vi "pathplan_vertices_send.vi"(1 "vertices":dbl[][](array[numeric]), 2 "distance_all":dbl, 4 "speed_max":dbl, 5 "写入串口":refnum<visa-resource-name>) -> (20 "路径规划数据写入缓冲区":string)   [LabVIEW 2016]
uses:
  <vilib>/imath/engines/lvmath2/RunTimeEngine/NodeEndStatement/NIMS_NodeEndStatement_Output.vi
  <instcachedir>/0/NIMS_NodeEndStatement_Output_53EC0D466D134D7ABD903AC30B43404B.lvgen/NIMS_NodeEndStatement_Output_53EC0D466D134D7ABD903AC30B43404B_011.vi
  <instcachedir>/0/NIMS_NodeEndStatement_Output_53EC0D466D134D7ABD903AC30B43404B.lvgen/NIMS_NodeEndStatement_Output_53EC0D466D134D7ABD903AC30B43404B_015.vi
  <vilib>/imath/engines/lvmath2/RunTimeEngine/ErrorHandling/NIMS_Finalize Error.vi
  <vilib>/imath/engines/lvmath2/RunTimeEngine/IndexRead/NIMS M($,S).vi
  <instcachedir>/0/NIMS M($,S)_3E5749BBB62E49528D4765A77F1F6D98.lvgen/NIMS M($,S)_3E5749BBB62E49528D4765A77F1F6D98_000.vi
  <vilib>/imath/engines/lvmath2/RunTimeEngine/ArithmeticOperatorToken/NIMS_ArithmeticOperator_minus.vi
  <instcachedir>/0/NIMS_ArithmeticOperator_minus_E3B65B1D26A44BB184AFDC5B3F458E3D.lvgen/NIMS_ArithmeticOperator_minus_E3B65B1D26A44BB184AFDC5B3F458E3D_017.vi
  <vilib>/imath/engines/lvmath2/RunTimeEngine/BuiltInFunctions/norm/NIMS_norm(GV,DBL).vi
  <instcachedir>/0/NIMS_norm(GV,DBL)_1268AFF3C646412B8C6EA3CE75D09042.lvgen/NIMS_norm(GV,DBL)_1268AFF3C646412B8C6EA3CE75D09042_000.vi
  <vilib>/imath/engines/lvmath2/RunTimeEngine/ErrorHandling/NIMS_Create Error From Enums.vi
  <vilib>/imath/engines/lvmath2/RunTimeEngine/RowToken/NIMS_RowToken_M_CV.vi
  <instcachedir>/0/NIMS_RowToken_M_CV_FA79F1D1D17D44459F3ED8E09EE8B625.lvgen/NIMS_RowToken_M_CV_FA79F1D1D17D44459F3ED8E09EE8B625_003.vi
  <vilib>/imathl/engines/lvmath/Functions/Error Handling/Create Error.vi
  <vilib>/imath/engines/lvmath2/RunTimeEngine/IndexRead/NIMS M($,R2).vi
  <instcachedir>/0/NIMS M($,R2)_D9380E19261A4ADFB2D364AF6959C6EF.lvgen/NIMS M($,R2)_D9380E19261A4ADFB2D364AF6959C6EF_001.vi
  <instcachedir>/0/NIMS_RowToken_M_CV_FA79F1D1D17D44459F3ED8E09EE8B625.lvgen/NIMS_RowToken_M_CV_FA79F1D1D17D44459F3ED8E09EE8B625_000.vi
  <vilib>/imath/engines/lvmath2/RunTimeEngine/BuiltInFunctions/size/NIMS_I32=size(GM,I32).vi
  <instcachedir>/0/NIMS_I32=size(GM,I32)_122058B1B3294FAEA5DC209B92B394E4.lvgen/NIMS_I32=size(GM,I32)_122058B1B3294FAEA5DC209B92B394E4_004.vi
  <vilib>/imath/engines/lvmath2/RunTimeEngine/RangeToken/NIMS_Range_R2 - Integer.vi
  <instcachedir>/0/NIMS_Range_R2 - Integer_89B873E74E6E489885E44F751DD9C6BF.lvgen/NIMS_Range_R2 - Integer_89B873E74E6E489885E44F751DD9C6BF_000.vi
  <vilib>/imath/engines/lvmath2/RunTimeEngine/CommandStatement/MC_CommandStatement_break.vi
  <instcachedir>/0/NIMS_ArithmeticOperator_minus_E3B65B1D26A44BB184AFDC5B3F458E3D.lvgen/NIMS_ArithmeticOperator_minus_E3B65B1D26A44BB184AFDC5B3F458E3D_003.vi
  <vilib>/imath/engines/lvmath2/RunTimeEngine/VariableToken/NIMS_VariableToken_CondDefined.vi
  <instcachedir>/0/NIMS_VariableToken_CondDefined_06E9DA95BD4D46A6BA55EC651A891960.lvgen/NIMS_VariableToken_CondDefined_06E9DA95BD4D46A6BA55EC651A891960_009.vi
  <vilib>/imath/engines/lvmath/Functions/Error Handling/MergeErrorsWrapper.vi
  <instcachedir>/0/NIMS_NodeEndStatement_Output_53EC0D466D134D7ABD903AC30B43404B.lvgen/NIMS_NodeEndStatement_Output_53EC0D466D134D7ABD903AC30B43404B_005.vi
  <instcachedir>/0/NIMS_NodeEndStatement_Output_53EC0D466D134D7ABD903AC30B43404B.lvgen/NIMS_NodeEndStatement_Output_53EC0D466D134D7ABD903AC30B43404B_010.vi
  <vilib>/imath/engines/lvmath2/RunTimeEngine/BuiltInFunctions/length/NIMS_length(GM).vi
  <instcachedir>/0/NIMS_length(GM)_47CEC356FCE0482D9BA47DC61C99F2C7.lvgen/NIMS_length(GM)_47CEC356FCE0482D9BA47DC61C99F2C7_000.vi
  <instcachedir>/0/NIMS_ArithmeticOperator_minus_E3B65B1D26A44BB184AFDC5B3F458E3D.lvgen/NIMS_ArithmeticOperator_minus_E3B65B1D26A44BB184AFDC5B3F458E3D_012.vi
  <vilib>/imath/engines/lvmath2/RunTimeEngine/IndexRead/NIMS V(S).vi
  <instcachedir>/0/NIMS V(S)_0488751826AF41519A22953C041130DC.lvgen/NIMS V(S)_0488751826AF41519A22953C041130DC_000.vi
  <instcachedir>/0/NIMS V(S)_0488751826AF41519A22953C041130DC.lvgen/NIMS V(S)_0488751826AF41519A22953C041130DC_002.vi
  <vilib>/imath/engines/lvmath2/RunTimeEngine/BuiltInFunctions/dot/NIMS_dot(GV,GV).vi
  <instcachedir>/0/NIMS_dot(GV,GV)_B9FAA411F4494E9B94D442721014A3FA.lvgen/NIMS_dot(GV,GV)_B9FAA411F4494E9B94D442721014A3FA_000.vi
  <instcachedir>/0/NIMS_NodeEndStatement_Output_53EC0D466D134D7ABD903AC30B43404B.lvgen/NIMS_NodeEndStatement_Output_53EC0D466D134D7ABD903AC30B43404B_009.vi
panel:
  out "队列中元素数量":i32
  out "元素":cluster{sgl, sgl, sgl, bool}
  out "vertices_set":i32[][](array[numeric])
  out "angle_send":dbl[](array[numeric])
  out "vertices_send":dbl[](array[numeric])
  out "speed_send":dbl[](array[numeric])
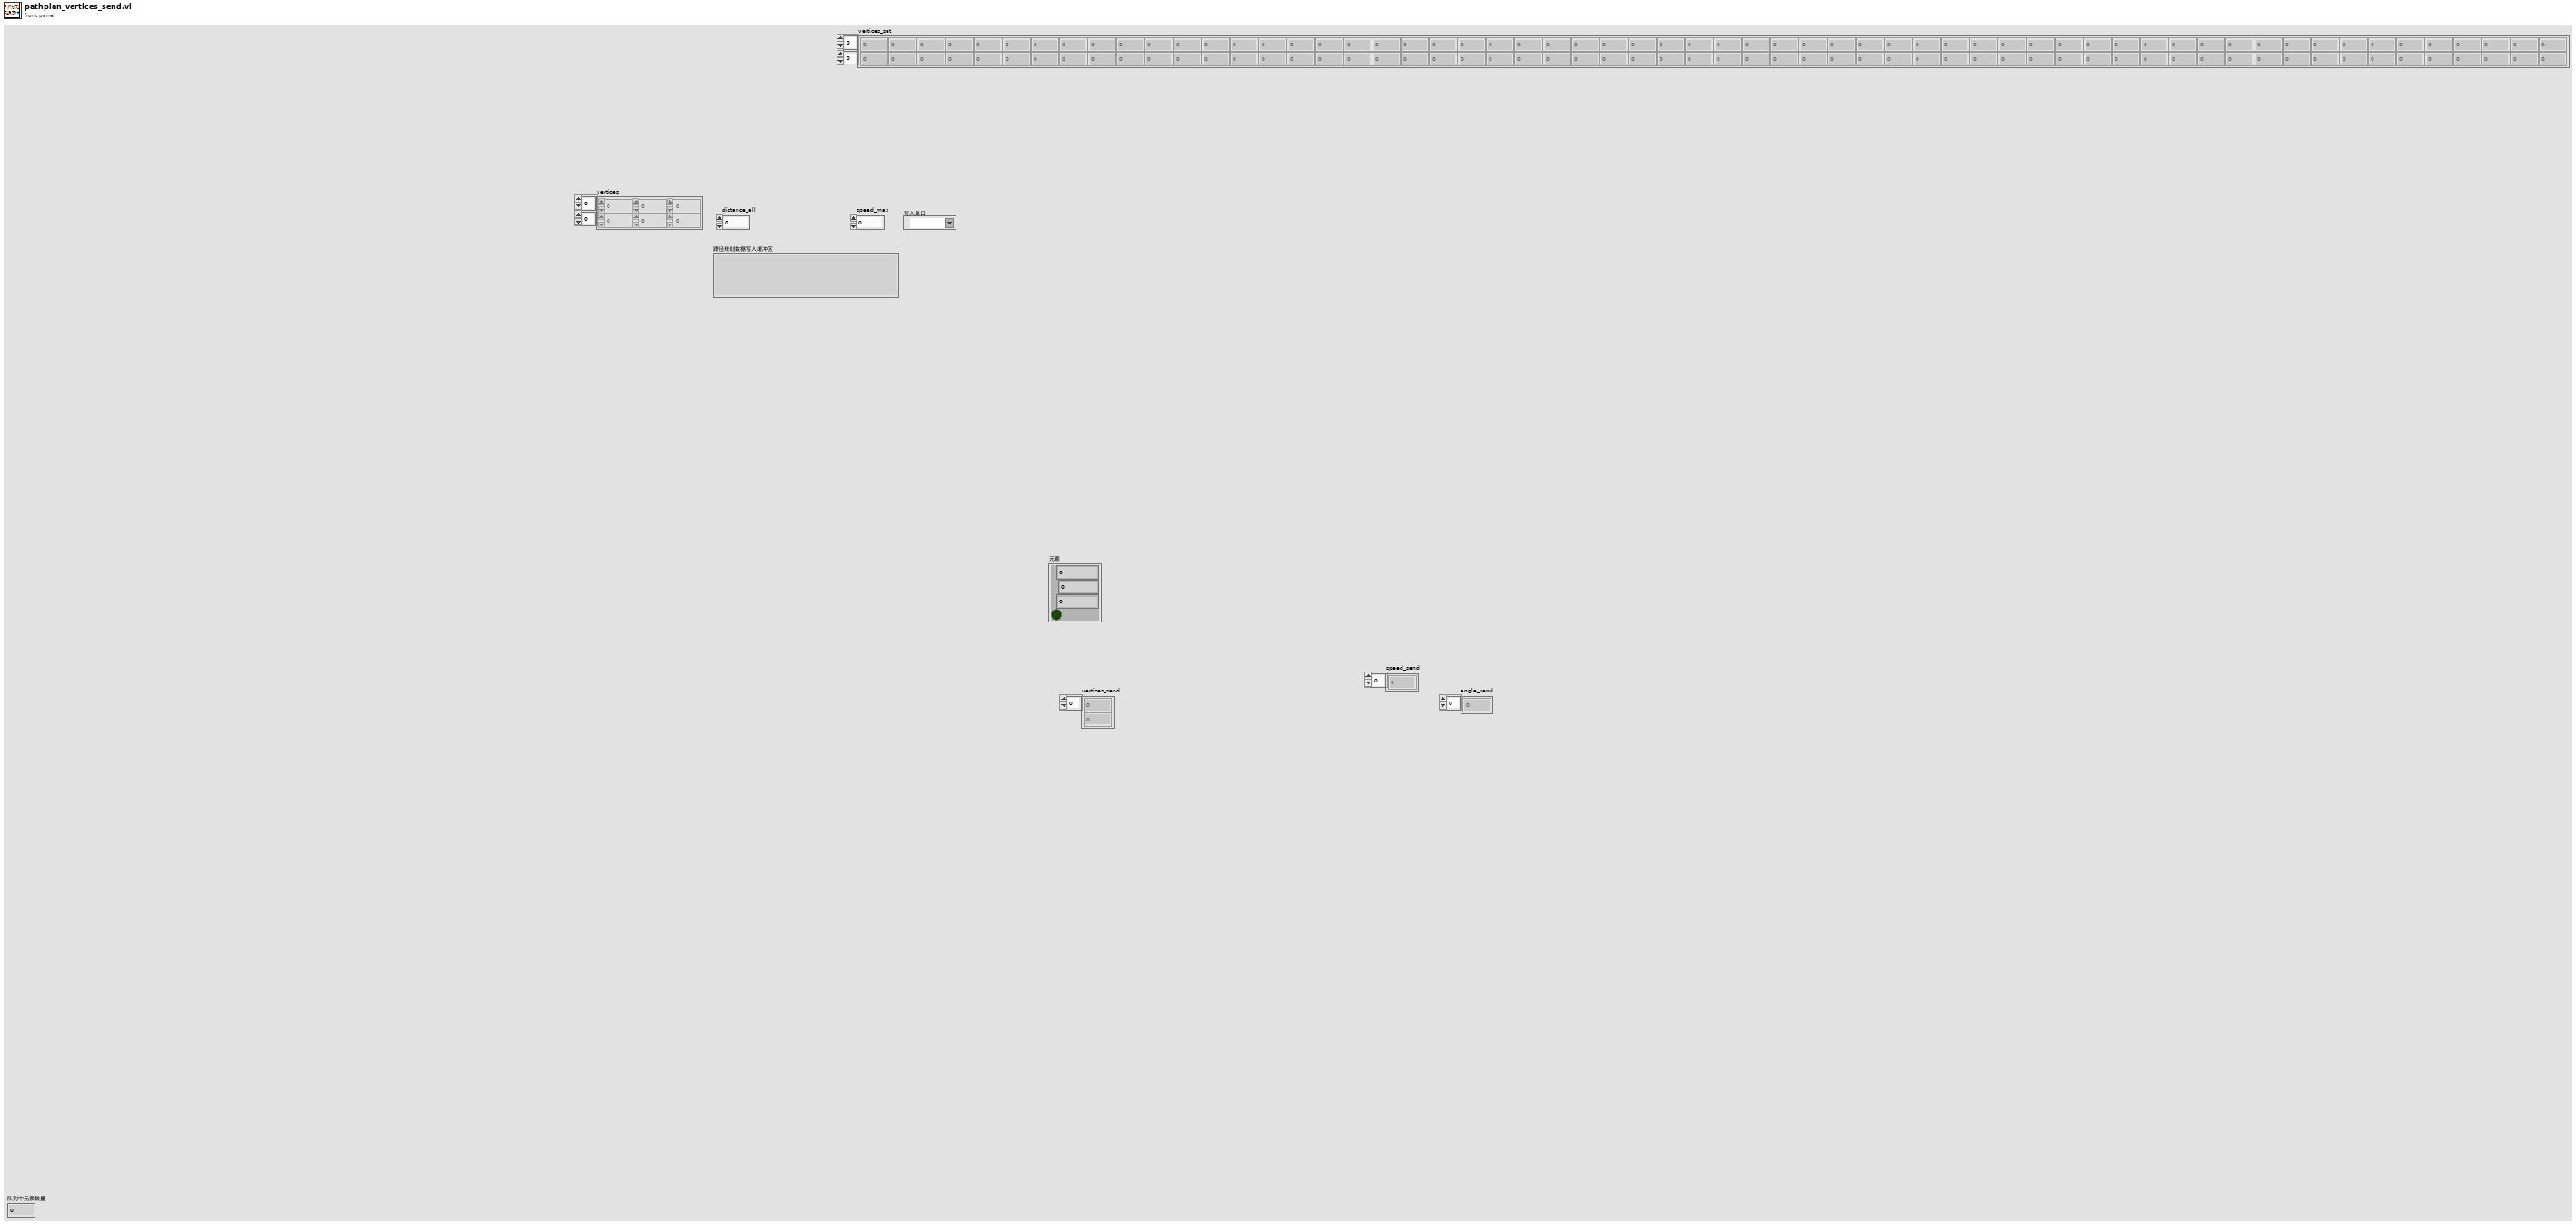
[diagram p1: front panel]
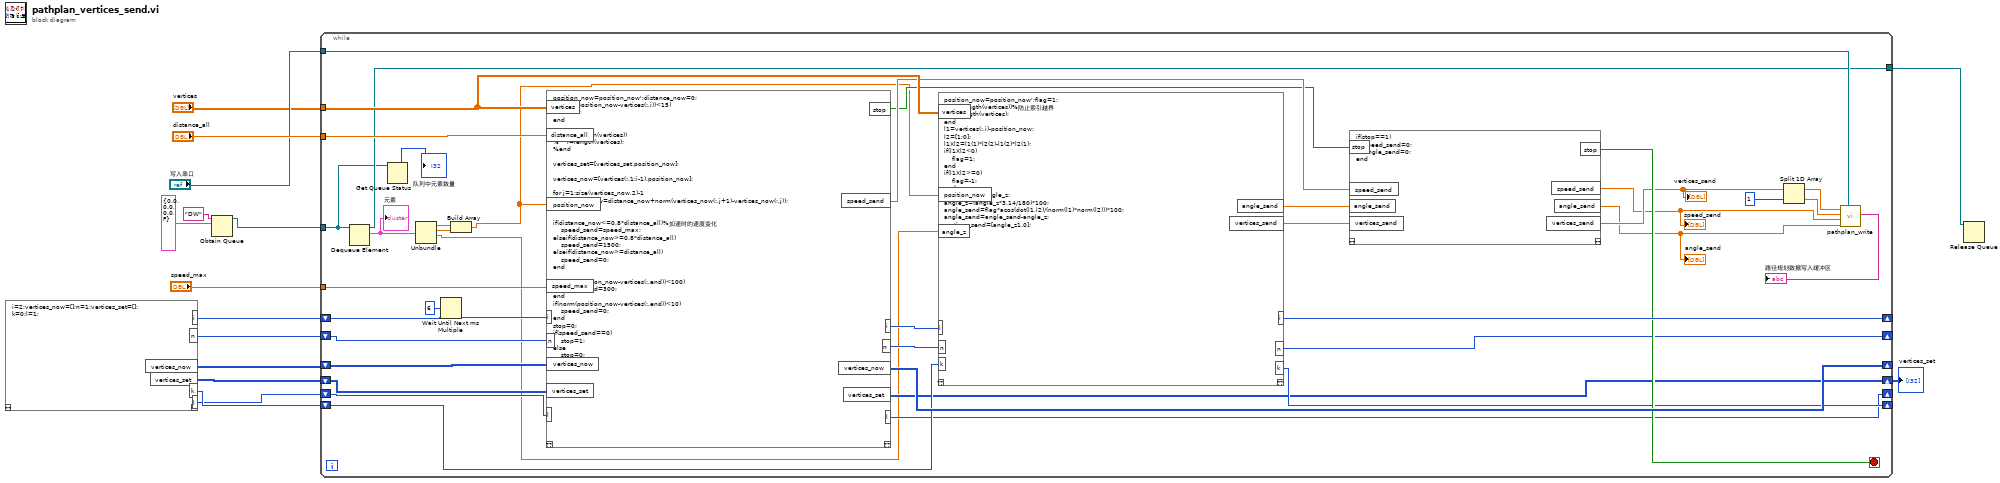
[diagram p0: block diagram]
diagram:
  n1 = mathscript code="i=2;vertices_now=[];n=1;vertices_set=[];\nk=0;l=1;"() -> ("i"=w14:i32, "vertices_now"=w12:i32[][], "n"=w9:i32, "vertices_set"=w7:i32[][], "k"=w8:i32, "l"=w6:i32)  [unwired: 1 in, 1 out]
  n2 = Obtain Queue(name (unnamed)="DW" ("名称（未命名）"), element data type=cluster{sgl, sgl, sgl, bool} {0.0, 0.0, 0.0, FALSE} ("输出簇 2")) -> (queue out=w2:refnum<queue>)  [unwired: 3 in, 2 out]
  n3 = while {
    tunnel: "vertices" -> [w53]
    tunnel: "distance_all" -> [w54]
    shift-right: [w52] -> _
    shift-left: w14 -> [w51]
    tunnel: "speed_max" -> [w50]
    shift-right: [w48] -> _
    shift-left: w12 -> [w34]
    tunnel: "写入串口" -> [w36]
    shift-right: [w31] -> _
    shift-left: w9 -> [w33]
    shift-right: [w29] -> _
    shift-left: w8 -> [w30]
    shift-right: [w25] -> w5
    shift-left: w7 -> [w28]
    shift-right: [w26] -> _
    shift-left: w6 -> [w27]
    tunnel: w2 -> [w16]
    tunnel: [w18] -> w1
    stop <- w40 stop-if-true
    n4 = Dequeue Element(queue=w16) -> (queue out=w18:refnum<queue>, element=w23:cluster{sgl, sgl, sgl, bool})  [unwired: 2 in, 2 out]
    "元素" <- w23
    n5 = Get Queue Status(queue=w16) -> (# elements in queue=→"队列中元素数量":i32)  [unwired: 2 in, 7 out]
    n6 = Unbundle(w23) -> (w22:sgl, w21:sgl, w19:sgl)  [unwired: 1 out]
    n7 = Wait Until Next ms Multiple(millisecond multiple=u32 6 ("毫秒倍数")) -> ()  [unwired: 1 out]
    n8 = Build Array(w22, w21) -> (w20:sgl[])
    n9 = mathscript code="position_now=position_now';distance_now=0;\nif(norm(position_now-vertices(:,i))<15)\n    i=i+1;\nend\n\n%if(i>=length(vertices))\n%    i=length(vertices);\n%end\n\nvertices_set=[vertices_set,position_now];\n\nvertices_now=[vertices(:,1:i-1),position_now];\n\nfor j=1:size(vertices_now,2)-1\n    distance_now=distance_now+norm(vertices_now(:,j+1)-vertices_now(:,j));\nend\n\nif(distance_now<=0.8*distance_all)%加速时的速度变化\n    speed_send=speed_max;\nelseif(distance_now>=0.8*distance_all)\n    speed_send=1500;\nelseif(distance_now>=distance_all)\n    speed_send=0;\nend\n\nif(norm(position_now-vertices(:,end))<100)\n    speed_send=300;\nend\nif(norm(position_now-vertices(:,end))<10)\n    speed_send=0;\nend\nstop=0;\nif(speed_send==0)\n    stop=1;\nelse\n    stop=0;\nend"("position_now"=w20, "vertices"=w53, "distance_all"=w54, "i"=w51, "speed_max"=w50, "vertices_now"=w34, "n"=w33, "vertices_set"=w28, "l"=w27) -> ("i"=w49:i32, "vertices_now"=w48:i32[][], "speed_send"=w43:dbl[], "stop"=w41:bool, "n"=w32:i32, "vertices_set"=w25:i32[][], "l"=w26:i32)  [unwired: 1 in, 1 out]
    n10 = mathscript code="position_now=position_now';flag=1;\nif(i>=length(vertices))%防止索引越界\n    i=length(vertices);\nend\nl1=vertices(:,i)-position_now;\nl2=[1;0];\nl1Xl2=l1(1)*l2(2)-l1(2)*l2(1);\nif(l1Xl2<0)\n    flag=1;\nend\nif(l1Xl2>=0)\n    flag=-1;\nend\nangle_z1=5*angle_z;\nangle_z=(angle_z*3.14/180)*100;\nangle_send=flag*acos(dot(l1,l2)/(norm(l1)*norm(l2)))*100;\nangle_send=angle_send-angle_z;\nvertices_send=[angle_z1,0];"("vertices"=w53, "position_now"=w20, "angle_z"=w19, "i"=w49, "n"=w32, "k"=w30) -> ("i"=w52:i32, "angle_send"=w44:cdb, "vertices_send"=w42:dbl[], "n"=w31:i32, "k"=w29:i32)  [unwired: 1 in, 1 out]
    n11 = mathscript code="if(stop==1)\n    speed_send=0;\n    angle_send=0;\nend"("speed_send"=w43, "angle_send"=w44, "vertices_send"=w42, "stop"=w41) -> ("stop"=w40:bool, "angle_send"=w37:dbl[], "speed_send"=w38:dbl[], "vertices_send"=w39:dbl[])  [unwired: 1 in, 1 out]
    "speed_send" <- w38
    "vertices_send" <- w39
    "angle_send" <- w37
    n12 = Split 1D Array(array=w39, index=1 ("索引")) -> (first subarray=w46:dbl[], second subarray=w45:dbl[])
    n13 = call "pathplan_write.vi"("VISA资源名称"=w36, "angle"=w37, "v"=w38, "y"=w45, "angle_err"=w46) -> ("路径规划数据写入缓冲区"=→"路径规划数据写入缓冲区":string)  [unwired: 6 in]
  }
  "vertices_set" <- w5
  n14 = Release Queue(queue=w1) -> ()  [unwired: 2 in, 3 out]
